vi "CRC_reflect.vi"(0 "CRC":u32 format="%.0x", 2 "Bits":u8, 5 "error in (no error)":errorcluster) -> (14 "Reflected CRC":u32 format="%.0x", 19 "error out":errorcluster)   [LabVIEW 2020]
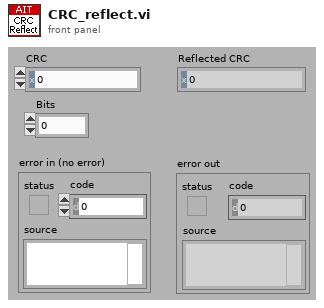
[diagram p1: front panel]
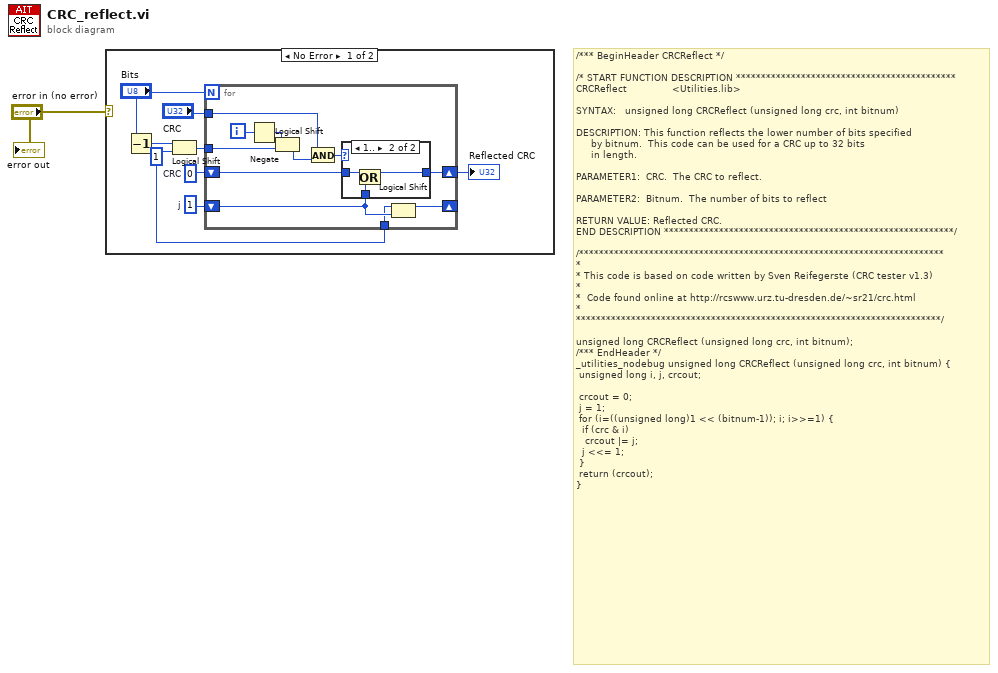
[diagram p0: block diagram]
diagram:
  # "/*** BeginHeader CRCReflect */\n\n/* START FUNCTION DESCRIPTION ********************************************\nCRCReflect\t\t\t\t\t\t\t\t\t\t\t\t\t\t\t<Utilities.lib>\n\nSYNTAX:\t\t\tunsigned long CRCReflect (unsigned long crc, int bitnum)\n\nDESCRIPTION:\tThis function reflects the lower number of bits specified\n\t\t\t\t\tby bitnum.  This code can be used for a CRC up to 32 bits\n\t\t\t\t\tin length.\n\nPARAMETER1:\t\tCRC.  The CRC to reflect.\n\nPARAMETER2:\t\tBitnum.  The number of bits to reflect\n\nRETURN VALUE:\tReflected CRC.\nEND DESCRIPTION **********************************************************/\n\n/*************************************************************************\n*\n*\tThis code is based on code written by Sven Reifegerste (CRC tester v1.3)\n*\n*  Code found online at http://rcswww.urz.tu-dresden.de/~sr21/crc.html\n*\n*************************************************************************/\n\nunsigned long CRCReflect (unsigned long crc, int bitnum);\n/*** EndHeader */\n_utilities_nodebug unsigned long CRCReflect (unsigned long crc, int bitnum) {\n\tunsigned long i, j, crcout;\n\n\tcrcout = 0;\n\tj = 1;\n\tfor (i=((unsigned long)1 << (bitnum-1)); i; i>>=1) {\n\t\tif (crc & i)\n\t\t\tcrcout |= j;\n\t\tj <<= 1;\n\t}\n\treturn (crcout);\n}"
  n1 = case shown="No Error" "error in (no error)" {
    frame No Error {
      w4 = u32 1  # j
      w3 = u32 1 ("x")
      w9 = u32 0  # CRC
      n2 = Decrement(x="Bits") -> (x-1=w5:u8)
      n3 = Logical Shift(y=w5, x=w3) -> (x << y=w2:u32)
      n4 = for {
        N: "Bits" -> [_]
        tunnel: "CRC" -> [w12]
        shift-right: [w19] -> w8
        shift-left: w9 -> [w18]
        shift-right: [w15] -> _
        shift-left: w4 -> [w14]
        tunnel: w3 -> [w13]
        tunnel: w2 -> [w10]
        i -> [w16]
        n5 = Negate(x=w16) -> (-x=w17:i32)
        n6 = Logical Shift(y=w17, x=w10) -> (x << y=w11:u32)
        n7 = And(x=w12, y=w11) -> (x .and. y?=w20:u32)
        n8 = case shown="1.." w20 {
          tunnel: w18 -> [w21 w24]
          tunnel: [w21 w23] -> w19
          tunnel: w14 -> [_ w22]
          frame ..0 {
          }
          frame 1.. {
            n9 = Or(x=w24, y=w22) -> (x .or. y?=w23:u32)
          }
        }
        n10 = Logical Shift(y=w13, x=w14) -> (x << y=w15:u32)
      }
      "Reflected CRC" <- w8
    }
    frame Error {
    }
  }
  "error out" <- "error in (no error)"
